vi "Add Analyzer.vi"(7 "Analyzer Subpanel":refnum<vi>, 8 "error in (no error)":errorcluster, 10 "new plugin":refnum<class "Generic Plugin.lvclass">, 11 "Plugin Array in":refnum<class "Controller Array.lvclass">) -> (0 "error out":errorcluster, 3 "Plugin Array out":refnum<class "Controller Array.lvclass">)   [LabVIEW 2020]
doc: "Adds a new analyzer plugin to the process cache."
uses:
  Controller/Generic Plugin.lvclass
  Controller Array/Controller Array.lvclass
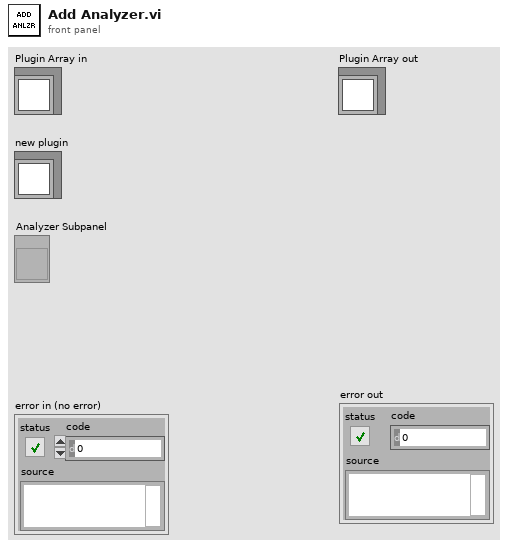
[diagram p1: front panel]
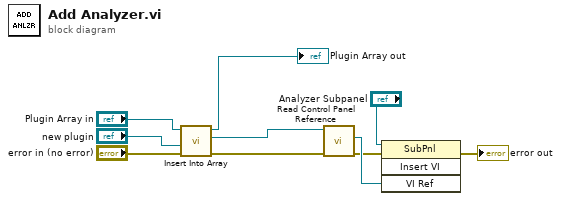
[diagram p0: block diagram]
diagram:
  n1 = call "Insert Into Array.vi"("error in (no error)"="error in (no error)", "new element"="new plugin", "Controller Array in"="Plugin Array in") -> ("error out"=w3:errorcluster, "new element"=w6:refnum<class "Generic Plugin.lvclass">, "Controller Array out"=→"Plugin Array out":refnum<class "Controller Array.lvclass">)  [unwired: 2 in]
  n2 = call "Read Control Panel Reference.vi"("error in (no error)"=w3, "controller in"=w6) -> ("error out"=w7:errorcluster, "Control Panel Reference"=w8:refnum<vi>)  [unwired: 7 in, 1 out]
  n3 = invoke on="Invoke Node" class="SubPnl" method="Insert VI"(reference="Analyzer Subpanel", error in=w7, "VI Ref"=w8) -> (error out=→"error out":errorcluster)  [unwired: 1 in, 3 out]
